vi "GPIB Error Report.vi"(2 "Function":string="A GPIB function ", 3 "Dialog?(F)":bool, 4 "Status":bool[](array[boolean])=[FALSE, FALSE, FALSE, FALSE, FALSE, FALSE, FALSE, FALSE, FALSE, FALSE, FALSE, FALSE, FALSE, FALSE, FALSE, FALSE], 5 "Address String":string) -> (0 "Error String":string, 1 "Status String":string)   [LabVIEW 2021]
doc: "Interpret the Status bits returned by a GPIB function and report the status and any error as text. If Dialog is True, the error message will be reported in a dialog box, and the user will have the choice of aborting or continuing."
panel:
  in  "Error strings":string[](array[string])=["NGER - No error to report", "ECIC - Command requires GPIB controller to be CIC", "ENOL - Write detected no listeners", "EADR - GPIB controller not addressed correctly", "EARG - Invalid argument or arguments", "ESAC - Command requires GPIB controller to be system controller", "EABO - I/O operation aborted", "ENEB - Non-existent board", "EDMA - DMA hardware error detected", "EBTO - DMA hardware uP bus timeout", "EOIP - New I/O attempted with old I/O in progress", "ECAP - No capability for operation", "EFSO - File system operation error", "EOWN - Sharable board exclusively owned", "TIMO - Timeout", "ESTB - Serial poll byte queue overflow", "ESRQ - SRQ stuck on", "ECMD - Unrecognized command", "", "EBNP - Board not present", "EINTRP - Interpreter error (MacBus)", "", "", "", "", "", "", "", "", "", "NADDR - No GPIB address input", "NSTRG - No string input (write)", "NCNT - No count input (read)", "", "", "", "", "", "", "", "EMOM - Out of memory (MacBus)", "EMIM - Insufficient memory (MacBus)", "", "", "", "", "", "", "", "", "ECOMM - Breakdown in SCSI protocols (MacBus)", "", "", "", "", "", "", "", "", "", "", "EPAR - Serial port parity error", "EORN - Serial port overrun error", "EOFL - Serial port receive buffer overflow", "EFRM - Serial port framing error", "SPTMO - Serial port timeout, bytes not received at serial port"]
  in  "Status bit strings":string[](array[string])=["DCAS - Device Clear State", "DTAS - Device Trigger State", "LACS - Listener Active State", "TACS - Talker Active State", "ATN - Attention Asserted", "CIC - Controller In Charge", "REM - Remote State", "LOK - Lockout State", "CMPL - Operation Completed", "", "", "", "SRQI - SRQ detected while CIC", "END - EOI or EOS detected", "TIMO - Timeout", "ERR - Error Detected"]
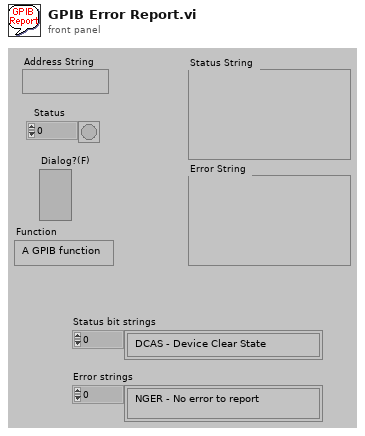
[diagram p1: front panel]
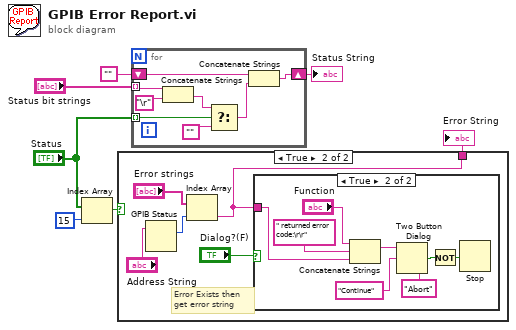
[diagram p0: block diagram]
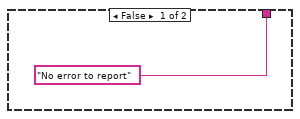
[diagram p2: hidden frame]
diagram:
  n1 = Index Array(array="Status", index=15) -> (element=w2:bool)
  n2 = case shown="True" w2 {
    tunnel: ["No error to report" w9] -> w1
    frame False {
    }
    frame True {
      # "Error Exists then get error string"
      n3 = GPIB Status(0:"Address String") -> (3:w11:i16)  [unwired: 1 in, 3 out]
      n4 = Index Array(array="Error strings", index=w11) -> (element=w9:string)
      n5 = case shown="True" "Dialog?(F)" {
        tunnel: w9 -> [_ w14]
        frame False {
        }
        frame True {
          n6 = Concatenate Strings("Function", " returned error code:\r\r", w14) -> (w20:string)
          n7 = Two Button Dialog(message=w20, 1:"Abort", 2:"Continue") -> (T button?=w17:bool)
          n8 = Not(x=w17) -> (.not. x?=w16:bool)
          n9 = Stop(stop? (T)=w16) -> ()
        }
      }
    }
  }
  "Error String" <- w1
  n10 = for {
    shift-right: [w22] -> w5
    shift-left: "" -> [w24]
    tunnel: "Status" -> [w27] mode=indexing
    tunnel: "Status bit strings" -> [w29] mode=indexing
    n11 = Concatenate Strings(w29, "\r") -> (w26:string)
    n12 = Select(t=w26, s=w27, f="") -> (s? t:f=w23:string)
    n13 = Concatenate Strings(w24, w23) -> (w22:string)
  }
  "Status String" <- w5
